vi "Create Request.vi"(5 "Request Type":T1, 7 "Room Number":i32, 8 "error in (no error)":errorcluster, 9 "Description":string, 10 "Name":string, 11 "Personnel Type":T2 items=["Nurse", "Doctor", "Cleanning", "Admin"]) -> (0 "error out":errorcluster, 2 "RUID":string, 3 "Request out":refnum<class "Request.lvclass">)   [LabVIEW 2015, in "Request.lvclass"]
uses:
  Request.lvclass
  PersonnelType.ctl
  RequestType.ctl
  Request.lvclass/Request.ctl
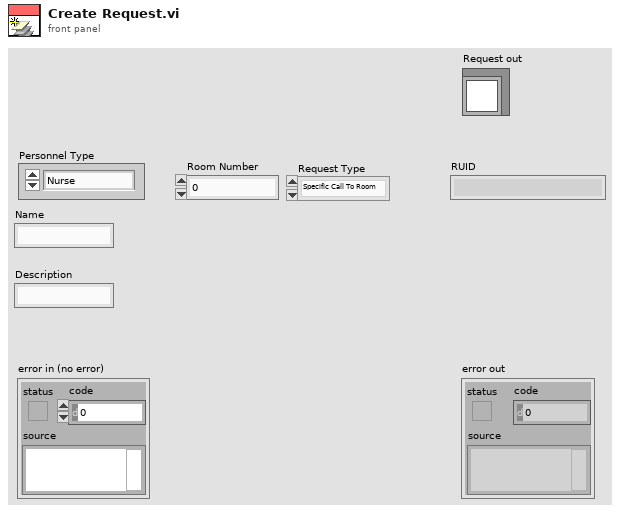
[diagram p1: front panel]
types:
  T1 = typedef "Request.lvclass/RequestType.ctl" = enum16{"Specific Call To Room", "General Call To Room"}
  T2 = typedef "Request.lvclass/PersonnelType.ctl" = u16
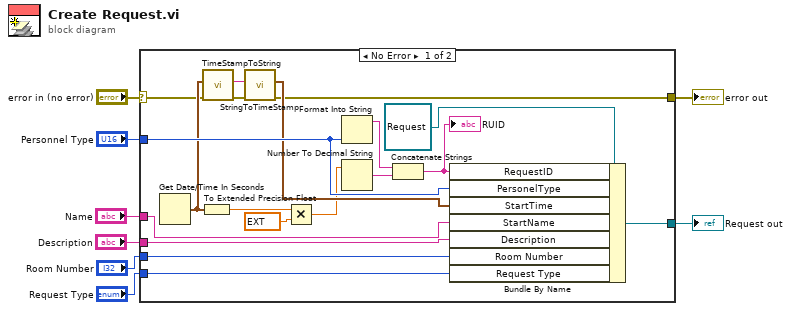
[diagram p0: block diagram]
diagram:
  n1 = case shown="No Error" "error in (no error)" {
    selector: "error in (no error)" -> [w18 w28]
    tunnel: [w16 w28] -> w7
    tunnel: [w27 _] -> w6
    tunnel: "Description" -> [w26 _]
    tunnel: "Name" -> [w25 _]
    tunnel: "Personnel Type" -> [w24 _]
    tunnel: "Room Number" -> [w15 _]
    tunnel: "Request Type" -> [w14 _]
    frame No Error {
      n2 = Get Date/Time In Seconds() -> (seconds since 1Jan1904=w21:timestamp)
      n3 = To Extended Precision Float(1:w21) -> (0:w12:ext)
      n4 = call "TimeStampToString.vi"("error in (no error)"=w18, "Time Stamp"=w21) -> ("error out"=w17:errorcluster, "String"=w20:string)  [unwired: 8 in]
      n5 = call "StringToTimeStamp.vi"("error in (no error)"=w17, "TimeStamp"=w20) -> ("error out"=w16:errorcluster, "Time Stamp"=w19:timestamp)  [unwired: 8 in]
      n6 = Multiply(x=w12, y=ext 10000.0) -> (x*y=w9:ext)
      n7 = Format Into String(w24) -> (resulting string=w23:string)  [unwired: 3 in, 1 out]
      n8 = Number To Decimal String(number=w9) -> (decimal integer string=w10:string)  [unwired: 1 in]
      n9 = Concatenate Strings(w23, w10) -> (w22:string)
      "RUID" <- w22
      n10 = Bundle By Name(cluster=refnum<class "Request.lvclass"> refnum ("Request in"), "RequestID"=w22, "PersonelType"=w24, "StartTime"=w19, "StartName"=w25, "Description"=w26, "Room Number"=w15, "Request Type"=w14) -> (w27:refnum<class "Request.lvclass">)
    }
    frame Error {
    }
  }
  "error out" <- w7
  "Request out" <- w6
